vi "sub_update_map-proviber.vi"() -> (0 "error out":errorcluster)   [LabVIEW 2019]
uses:
  C:/Users/WEGO/Documents/GitHub/Ycar/LabVIEW/Gmap/dll/GMap.NET.Core.dll
  dll/GMap.NET.Core.dll
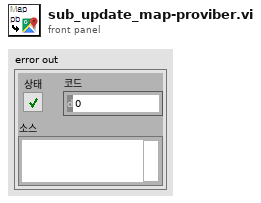
[diagram p1: front panel]
types:
  T1 = typedef "mapinfo.ctl" = cluster{"GmapDotNet":refnum<k24>, "mapprovider_info":cluster{"index":i32, "dotnetrefs":refnum<k24>, "Name":string}[]}
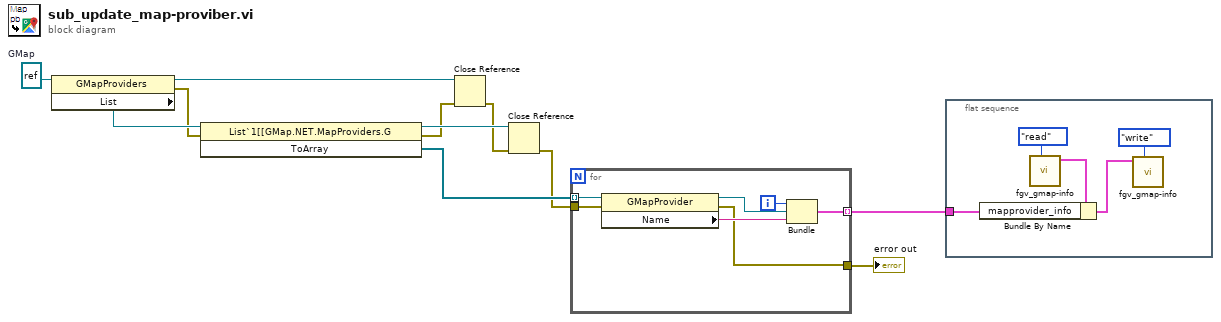
[diagram p0: block diagram]
diagram:
  w9 = refnum<k24> refnum  # GMap
  n1 = property class="GMapProviders"(reference=w9) -> (reference out=w7:refnum<k24>, error out=w6:errorcluster, "List"=w10:refnum<k24>)  [unwired: 1 in]
  n2 = invoke class="List`1[[GMap.NET.MapProviders.G" method="ToArray"(reference=w10, error in=w6) -> (reference out=w8:refnum<k24>, error out=w5:errorcluster, "ToArray"=w11:refnum<k24>[])  [unwired: 1 in]
  n3 = Close Reference(reference=w7, error in (no error)=w5) -> (error out=w4:errorcluster)
  n4 = Close Reference(reference=w8, error in (no error)=w4) -> (error out=w2:errorcluster)
  n5 = for {
    tunnel: w11 -> [w16] mode=indexing
    tunnel: [w15] -> w3 mode=indexing
    tunnel: w2 -> [w13]
    tunnel: [w12] -> w1
    i -> [w17]
    n6 = property class="GMapProvider"(reference=w16, error in=w13) -> (reference out=w14:refnum<k24>, error out=w12:errorcluster, "Name"=w18:string)
    n7 = Bundle(w17, w14, "Name"=w18) -> (w15:cluster{i32, refnum<k24>, "Name":string})  [unwired: 1 in]
  }
  "error out" <- w1
  n8 = flat-sequence {
    tunnel: w3 -> [w19]
    frame #0 {
      n9 = call "fgv_gmap-info.vi"("cmd"=enum16{"read", "write"}."read") -> ("mapinfo 2"=w22:T1)  [unwired: 9 in, 1 out]
      n10 = Bundle By Name(cluster=w22, "mapprovider_info"=w19) -> (w20:T1)
      n11 = call "fgv_gmap-info.vi"("cmd"=enum16{"read", "write"}."write", "mapinfo"=w20) -> ()  [unwired: 8 in, 2 out]
    }
  }
